vi "Excel Report - Conditionally Formatted Spreadsheet.vi"() -> ()   [LabVIEW 2023]
doc: "This example creates a new workbook, inserts a numerical table and calls the Excel Set Cell Format VI to customize the cell number format. \n\nThe VI formats the used section of the spreadsheet so that values lower than 0.5 display in blue, and the values greater than 0.5 display in red.\n\nRefer to the Excel documentation for more information about number format."
uses:
  <vilib>/Utility/NIReport.llb/Report Type.ctl
  <vilib>/Utility/NIReport.llb/Append Numeric Table to Report (wrap).vi
  <vilib>/Utility/NIReport.llb/NI_report.lvclass
  <vilib>/Utility/NIReport.llb/Excel/NI_Excel.lvclass
  <vilib>/Utility/NIReport.llb/NI_ReportGenerationCore.lvlib
panel:
  in  "Format":string="[Red][<=0.5];[Blue][>0.5]"
  # "Overview: This example creates a new workbook, inserts a numerical table, and calls the Excel Set Cell Format VI in order to customize the cell number format. \nRequirements: Report Generation Toolkit, Microsoft Excel\nInstructions:\nRun the VI and observe the building of the Excel spreadsheet.\n\n\nNote: \nRefer to the Excel documentation for more information about number formats. \nIf you are using a non English version of Microsoft Excel, you need to change the colors in this string to language-specific."
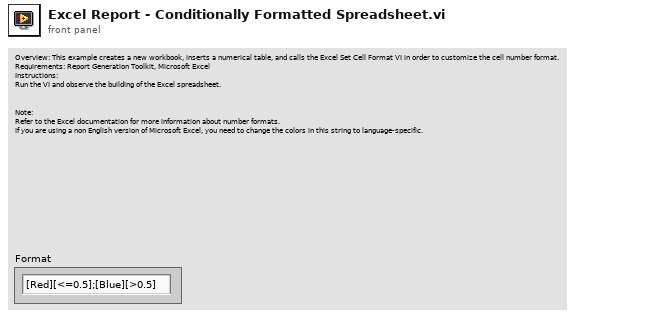
[diagram p1: front panel]
types:
  T1 = typedef "NI_ReportGenerationCore.lvlib/Report Type.ctl" = enum16{"HTML", "Word", "Excel"}
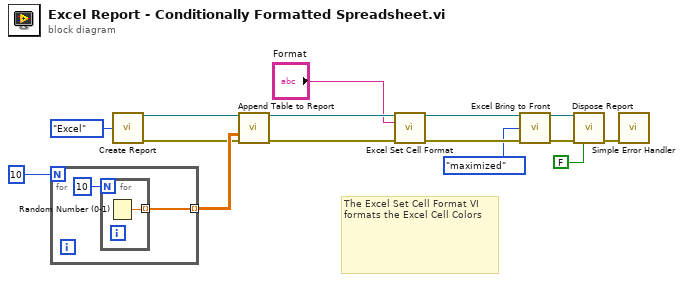
[diagram p0: block diagram]
diagram:
  # "The Excel Set Cell Format VI formats the Excel Cell Colors"
  n1 = for {
    N: 10 -> [_]
    tunnel: [w17] -> w15 mode=indexing
    n2 = for {
      N: 10 ("dimension size") -> [_]
      tunnel: [w18] -> w17 mode=indexing
      n3 = Random Number (0-1)() -> (number: 0 to 1=w18:dbl)
    }
  }
  n4 = call <vilib>:"Create Report.vi"("report type"=Report_Type."Excel" ("Report Type")) -> ("report out"=w13:refnum<class "NI_report.lvclass">, "error out"=w14:errorcluster)  [unwired: 13 in]
  n5 = call-poly <vilib>:"Append Table to Report.vi"("report in"=w13, "numerical data"=w15, "error in (no error)"=w14) -> ("report out"=w11:refnum<class "NI_report.lvclass">, "error out"=w12:errorcluster)  [unwired: 9 in, 2 out]
  n6 = call <vilib>:"Excel Set Cell Format.vi"("report in"=w11, "number format"="Format", "error in (no error)"=w12) -> ("report out"=w7:refnum<class "NI_report.lvclass">, "error out"=w8:errorcluster)  [unwired: 11 in]
  n7 = call <vilib>:"Excel Bring to Front.vi"("report in"=w7, "window state (maximized)"=enum16{"maximized", "minimized", "normal"}."maximized", "error in (no error)"=w8) -> ("report out"=w3:refnum<class "NI_report.lvclass">, "error out"=w5:errorcluster)  [unwired: 11 in]
  n8 = call-dynamic "Dispose Report.vi"("report in"=w3, "error in (no error)"=w5, "close report? (T)"=FALSE ("Close Report? (T)")) -> ("error out"=w4:errorcluster)  [unwired: 12 in]
  n9 = call <vilib>:"Simple Error Handler.vi"("error in (no error)"=w4) -> ()  [unwired: 4 in, 5 out]
